vi "comparitive 5.vi"() -> ()   [LabVIEW 2025]
panel:
  out "Boolean 2":bool
  out "Boolean":bool
  out "c":dbl
  in  "b":dbl
  in  "a":dbl
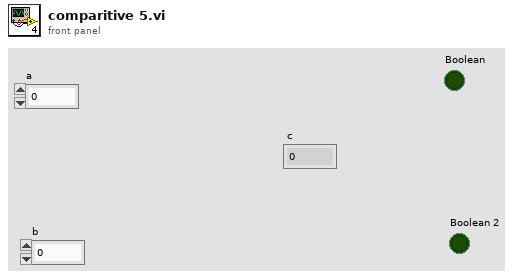
[diagram p1: front panel]
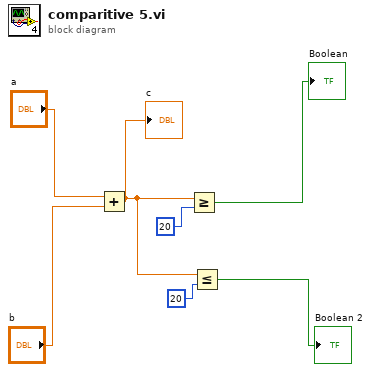
[diagram p0: block diagram]
diagram:
  n1 = Add(x="a", y="b") -> (x+y=w1:dbl)
  "c" <- w1
  n2 = Greater Or Equal?(x=w1, y=20) -> (x >= y?=→"Boolean":bool)
  n3 = Less Or Equal?(x=w1, y=20) -> (x <= y?=→"Boolean 2":bool)
